vi "main.vi"() -> ()   [LabVIEW 2017]
uses:
  <vilib>/DAQmx/read.llb/DAQmx Read.vi
  <vilib>/DAQmx/read.llb/DAQmx Read (Analog 1D Wfm NChan NSamp).vi
  <vilib>/DAQmx/create/channels.llb/DAQmx Create Channel (AI-Voltage-Basic).vi
  <vilib>/DAQmx/create/channels.llb/DAQmx Create Channel (AI-Current-Basic).vi
  <vilib>/DAQmx/configure/timing.llb/DAQmx Timing (Sample Clock).vi
  <vilib>/DAQmx/miscellaneous.llb/DAQmx Fill In Error Info.vi
panel:
  out "Waveform Chart 3":waveform(dbl)(graph)
  out "Waveform Chart 2":waveform(dbl)(graph)
  out "Waveform Chart":waveform(dbl)(graph)
  in  "stop":bool
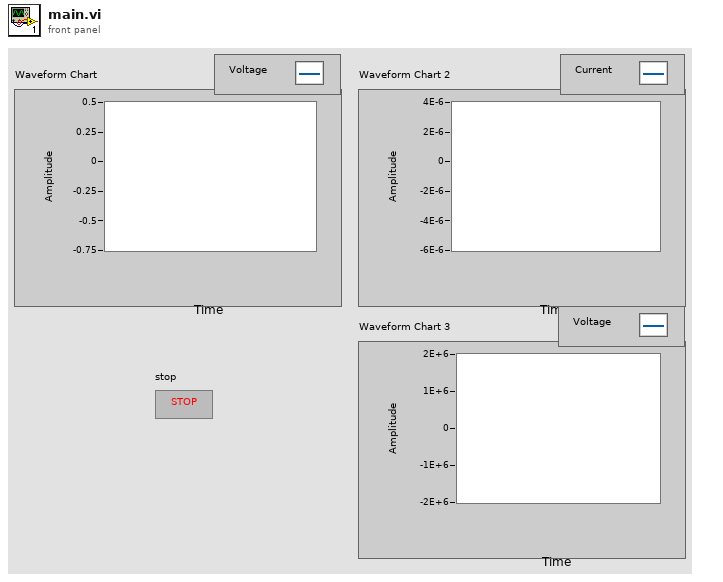
[diagram p1: front panel]
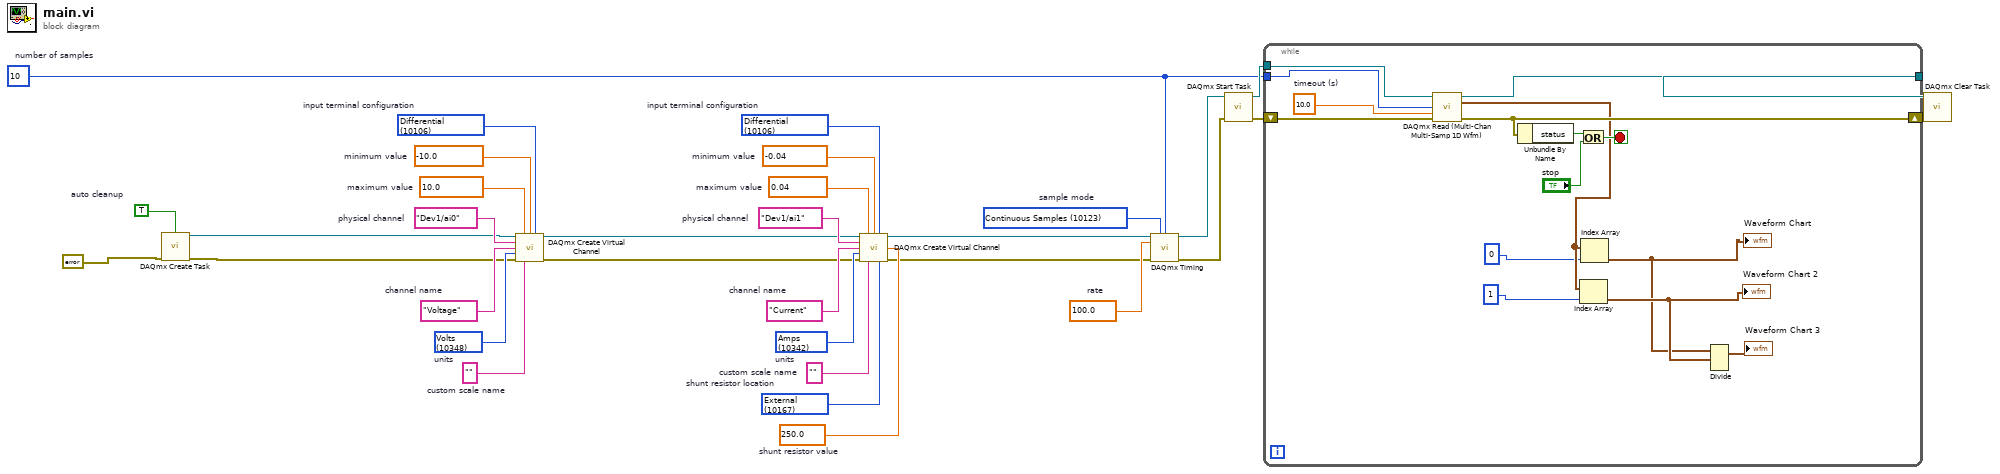
[diagram p0: block diagram]
diagram:
  w27 = 10123 items=["Finite Samples"=10178, "Continuous Samples"=10123, "Hardware Timed Single Point"=12522]  # sample mode
  w26 = 100.0  # rate
  w24 = 10106 items=["default"=-1, "RSE"=10083, "NRSE"=10078, "Differential"=10106, "Pseudodifferential"=12529]  # input terminal configuration
  w23 = 10342 items=["Amps"=10342, "From Custom Scale"=10065]  # units
  w22 = 250.0  # shunt resistor value
  w21 = 10167 items=["Internal"=10200, "External"=10167]  # shunt resistor location
  w20 = "Current"  # channel name
  w18 = ""  # custom scale name
  w17 = -0.04  # minimum value
  w16 = 0.04  # maximum value
  w15 = "Dev1/ai1"  # physical channel
  w13 = 10106 items=["default"=-1, "RSE"=10083, "NRSE"=10078, "Differential"=10106, "Pseudodifferential"=12529]  # input terminal configuration
  w12 = 10348 items=["Volts"=10348, "From Custom Scale"=10065]  # units
  w11 = "Voltage"  # channel name
  w9 = ""  # custom scale name
  w8 = -10.0  # minimum value
  w7 = 10.0  # maximum value
  w6 = "Dev1/ai0"  # physical channel
  w4 = TRUE  # auto cleanup
  w1 = 10  # number of samples
  n1 = call <vilib>:"DAQmx Create Task.vi"("auto cleanup"=w4, "error in"=errorcluster {"status"=FALSE, "code"=0, "source"=""}) -> ("task out"=w5:refnum<k21>, "error out"=w3:errorcluster)  [unwired: 12 in]
  n2 = call-poly <vilib>:"DAQmx Create Virtual Channel.vi"("task in"=w5, "maximum value"=w7, "minimum value"=w8, "input terminal configuration"=w13, "physical channels"=w6, "name to assign"=w11, "units"=w12, "error in"=w3, "custom scale name"=w9) -> ("task out"=w14:refnum<k21>, "error out"=w10:errorcluster)  [unwired: 5 in]
  n3 = call-poly <vilib>:"DAQmx Create Virtual Channel.vi"("task in"=w14, "maximum value"=w16, "minimum value"=w17, "input terminal configuration"=w24, "physical channels"=w15, "name to assign"=w20, "external shunt resistor value"=w22, "units"=w23, "error in"=w10, "custom scale name"=w18, "shunt resistor location"=w21) -> ("task out"=w25:refnum<k21>, "error out"=w19:errorcluster)  [unwired: 3 in]
  n4 = call-poly <vilib>:"DAQmx Timing.vi"("task/channels in"=w25, "sample mode"=w27, "samples per channel"=w1, "rate"=w26, "error in"=w19) -> ("task out"=w2:refnum<k21>, "error out"=w29:errorcluster)  [unwired: 9 in]
  n5 = call <vilib>:"DAQmx Start Task.vi"("task/channels in"=w2, "error in"=w29) -> ("task out"=w33:refnum<k21>, "error out"=w32:errorcluster)  [unwired: 12 in]
  n6 = while {
    tunnel: w33 -> [w48]
    tunnel: w1 -> [w45]
    tunnel: [w46] -> w30
    shift-right: [w43] -> w31
    shift-left: w32 -> [w47]
    stop <- w42 stop-if-true
    w40 = 10.0  # timeout (s)
    n7 = call-poly "DAQmx Read (Multi-Chan Multi-Samp 1D Wfm).vi"("task/channels in"=w48, "number of samples per channel"=w45, "timeout"=w40, "error in"=w47) -> ("task out"=w46:refnum<k21>, "data"=w39:waveform(dbl)[], "error out"=w43:errorcluster)  [unwired: 9 in]
    n8 = Unbundle By Name(w43) -> ("status"=w44:bool)
    n9 = Or(x=w44, y="stop") -> (x .or. y?=w42:bool)
    n10 = Index Array(array=w39, index=1) -> (element=w38:waveform(dbl))
    "Waveform Chart 2" <- w38
    n11 = Index Array(array=w39, index=0) -> (element=w36:waveform(dbl))
    "Waveform Chart" <- w36
    n12 = Divide(1:w38, 2:w36) -> (0:→"Waveform Chart 3":waveform(dbl))  [unwired: 1 in, 1 out]
  }
  n13 = call <vilib>:"DAQmx Clear Task.vi"("task in"=w30, "error in"=w31) -> ()  [unwired: 13 in, 1 out]
